vi "Get Command Info from library.vi"(9 "Step":string, 10 "Imported Commands":string[][](array[string])) -> (3 "Data cluster":T1)   [LabVIEW 2020]
uses:
  Data Cluster.ctl
  3ce336a9-9f4b-4c7f-adf6-01c178456532.vi
  <vilib>/Comparison/Equal/Equal Functor/Equal Functor.lvclass
panel:
  # "Send Data:"
  # "Receive Data:"
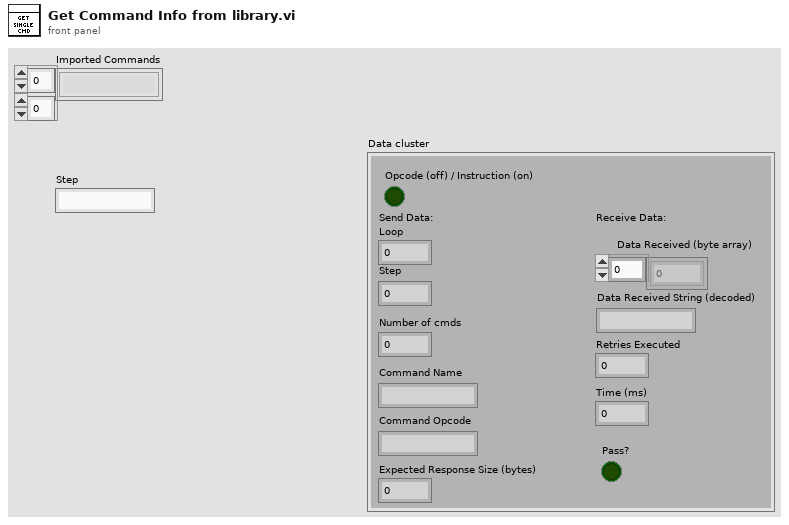
[diagram p1: front panel]
types:
  T1 = typedef "Data Cluster.ctl" = cluster{"Command Name":string, "Command Opcode ":string, "Step":dbl, "Loop":dbl, "Expected Response Size (bytes)":u16, "Number of cmds":dbl, "Data Received (byte array)":u8[], "Retries Executed":u16, "Time (ms)":u16, "Pass?":bool, "Opcode (off) / Instruction (on)":bool, "Data Received String (decoded)":string}
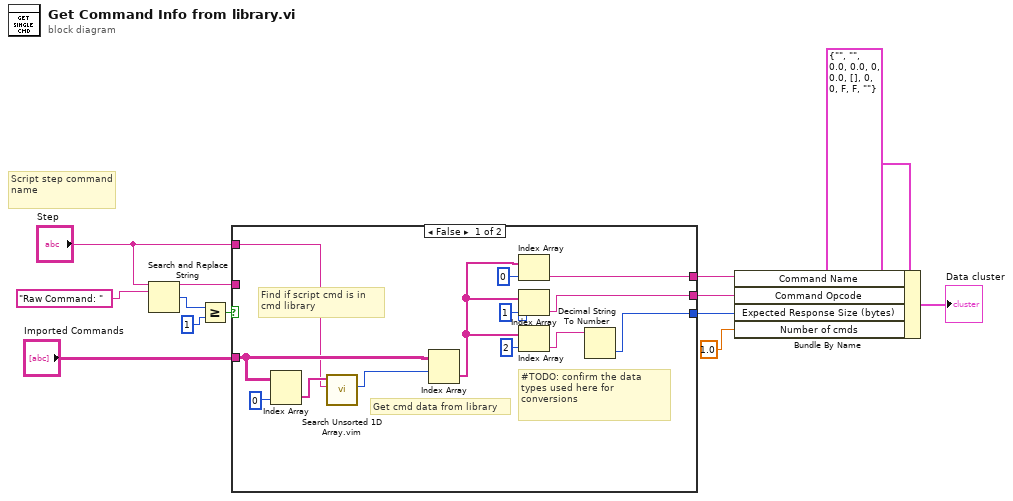
[diagram p0: block diagram]
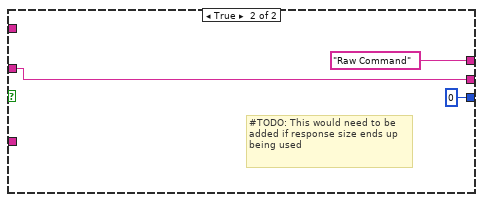
[diagram p2: hidden frame]
diagram:
  # "Script step command name"
  n1 = Search and Replace String(input string="Step", search string="Raw Command: ") -> (result string=w7:string, number of replacements=w10:i32)  [unwired: 6 in, 2 out]
  n2 = Greater Or Equal?(x=w10, y=1) -> (x >= y?=w8:bool)
  n3 = case shown="False" w8 {
    tunnel: w7 -> [_ w28]
    tunnel: "Imported Commands" -> [w21 _]
    tunnel: "Step" -> [w14 _]
    tunnel: [w19 "Raw Command"] -> w4
    tunnel: [w17 0] -> w5
    tunnel: [w16 w28] -> w3
    frame False {
      # "#TODO: confirm the data types used here for conversions"
      # "Get cmd data from library"
      # "Find if script cmd is in cmd library"
      n4 = Index Array(array=w21, index (col)=0 ("disabled index (col)")) -> (element=w15:string[])  [unwired: 1 in]
      n5 = call "Search Unsorted 1D Array.vim"("element"=w14, "unsorted 1D array"=w15) -> ("index of element"=w26:i32)  [unwired: 9 in]
      n6 = Index Array(array=w21, index (row)=w26) -> (element=w20:string[])  [unwired: 1 in]
      n7 = Index Array(array=w20, index=0) -> (element=w19:string)
      n8 = Index Array(array=w20, index=1) -> (element=w16:string)
      n9 = Index Array(array=w20, index=2) -> (element=w18:string)
      n10 = Decimal String To Number(string=w18) -> (number=w17:i32)  [unwired: 2 in, 1 out]
    }
    frame True {
      # "#TODO: This would need to be added if response size ends up being used"
    }
  }
  n11 = Bundle By Name(cluster=T1 {"Command Name"="", "Command Opcode "="", "Step"=0.0, "Loop"=0.0, "Expected Response Size (bytes)"=0, "Number of cmds"=0.0, "Data Received (byte array)"=[], "Retries Executed"=0, "Time (ms)"=0, "Pass?"=FALSE, "Opcode (off) / Instruction (on)"=FALSE, "Data Received String (decoded)"=""} ("Data Cluster"), "Command Name"=w4, "Command Opcode"=w3, "Expected Response Size (bytes)"=w5, "Number of cmds"=1.0) -> (→"Data cluster":T1)
